vi "Get All Paths.vi"(4 "is array element?":bool, 6 "index string":string, 8 "error in (no error)":errorcluster, 9 "parents":string[](array[string]), 10 "Variant":variant, 11 "Paths":string[](array[string])) -> (0 "error out":errorcluster, 3 "Paths out":string[](array[string]))   [LabVIEW 2017, in "Advanced Variant Tools.lvlib"]
uses:
  Advanced Variant Tools.lvlib
  <vilib>/Utility/Data Type/NI_Data Type.lvlib
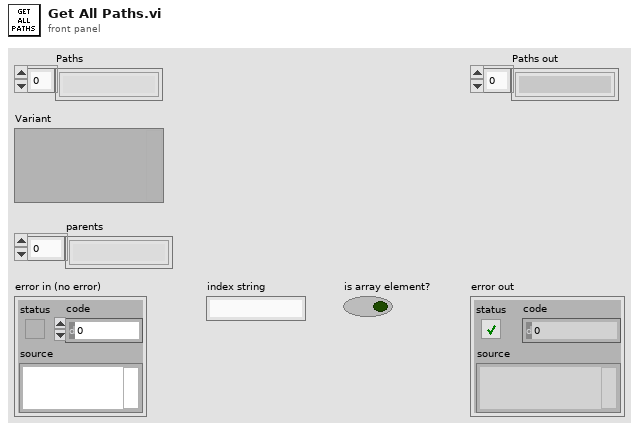
[diagram p1: front panel]
types:
  T1 = typedef "NI_Data Type.lvlib/Data Type.ctl" = enum8{"Invalid Type", "Void", "I8", "I16", "I32", "I64", "U8", "U16", "U32", "U64", "Single Float", "Double Float", "Extended Float", "Single Complex", "Double Complex", "Extended Complex", "Enum U8", "Enum U16", "Enum U32", "Enum U64", "Single Float With Unit", "Double Float With Unit", "Extended Float With Unit", "Single Complex with Unit", "Double Complex with Unit", "Extended Complex with Unit", "Boolean", "String", "Path", "Picture", "Tag", "Array", "Cluster", "Variant", "LV Variant", "Waveform", "Timestamp", "Digital Waveform", "Digital Data", "ExpressData", "Refnum", "External Data", "VI", "Poly VI", "LabVIEW Class Instance", "Fixed Point"}
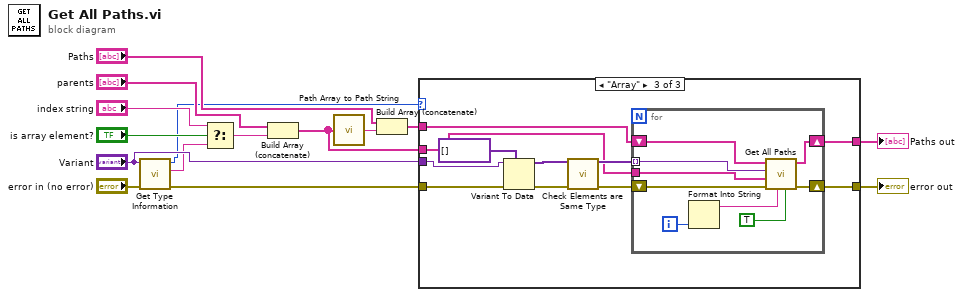
[diagram p0: block diagram]
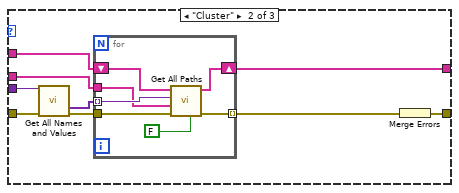
[diagram p3: hidden frame]
diagram:
  n1 = call <vilib>:"Get Type Information.vi"("error in (no error)"="error in (no error)", "Variant"="Variant") -> ("error out"=w15:errorcluster, "Name"=w1:string, "Type"=w2:T1)  [unwired: 5 in, 2 out]
  n2 = Select(t="index string", s="is array element?", f=w1) -> (s? t:f=w9:string)
  n3 = Build Array (concatenate)("parents", w9) -> (w8:string[])
  n4 = call "Path Array to Path String.vi"("path array"=w8) -> ("path"=w5:string)  [unwired: 14 in]
  n5 = Build Array (concatenate)("Paths", w5) -> (w4:string[])
  n6 = case shown="\"Array\"" w2 {
    tunnel: w15 -> [w17 w19 w40]
    tunnel: [w17 w23 w44] -> w10
    tunnel: "Variant" -> [_ w26 w42]
    tunnel: w8 -> [_ w22 w36]
    tunnel: w4 -> [w16 w21 w35]
    tunnel: [w16 w20 w34] -> w3
    frame Default {
    }
    frame "Cluster" {
      n7 = call "Get All Names and Values.vi"("Variant (Cluster) In"=w26, "error in"=w19) -> ("Values"=w25:variant[], "error out"=w18:errorcluster)  [unwired: 9 in, 3 out]
      n8 = for {
        tunnel: w25 -> [w33] mode=indexing
        tunnel: [w32] -> w24 mode=indexing
        shift-right: [w27] -> w20
        shift-left: w21 -> [w28]
        tunnel: w18 -> [w30]
        tunnel: w22 -> [w29]
        n9 = call "Get All Paths.vi"("is array element?"=FALSE ("first call?"), "error in (no error)"=w30, "parents"=w29, "Variant"=w33, "Paths"=w28) -> ("error out"=w32:errorcluster, "Paths out"=w27:string[])  [unwired: 5 in]
      }
      n10 = Merge Errors(w24) -> (w23:errorcluster)
    }
    frame "Array" {
      n11 = Variant To Data(error in=w40, type=variant[] [], Variant=w42) -> (data=w41:variant[], error out=w39:errorcluster)
      n12 = call "Check Elements are Same Type.vi"("array in"=w41, "error in (no error)"=w39) -> ("array out"=w38:variant[], "error out"=w37:errorcluster)  [unwired: 12 in]
      n13 = for {
        tunnel: w38 -> [w50] mode=indexing
        shift-right: [w53] -> w44
        shift-left: w37 -> [w52]
        shift-right: [w46] -> w34
        shift-left: w35 -> [w45]
        tunnel: w36 -> [w47]
        i -> [w49]
        n14 = Format Into String(w49) -> (resulting string=w48:string)  [unwired: 3 in, 1 out]
        n15 = call "Get All Paths.vi"("is array element?"=TRUE ("first call?"), "index string"=w48, "error in (no error)"=w52, "parents"=w47, "Variant"=w50, "Paths"=w45) -> ("error out"=w53:errorcluster, "Paths out"=w46:string[])  [unwired: 4 in]
      }
    }
  }
  "error out" <- w10
  "Paths out" <- w3
